vi "Load_Portfolio.vi"(7 "Config File path":path caption="Config File Path", 8 "error in (no error)":errorcluster caption="entrée d'erreur (pas d'erreur)", 11 "path":path) -> (0 "error out":errorcluster caption="sortie d'erreur", 3 "Portfolio en sortie":refnum<class "Portfolio.lvclass"> caption="DNL_LabVIEW Object out")   [LabVIEW 2012, in "Portfolio.lvclass"]
uses:
  Portfolio.lvclass
  Portfolio.lvclass/Portfolio.ctl
  Operation/Operation Parameters.ctl
  Operation/Operation Type Enum.ctl
  controls/Currencies.ctl
  Operation/Operation.lvclass
  Operation/Operation.lvclass/Operation.ctl
  Exchange/Exchange Parameters.ctl
  Exchange/Exchange Type Enum.ctl
  Exchange/Exchange.lvclass
  Exchange/Exchange.lvclass/Exchange.ctl
  Operations/Operations.lvclass
  Exchanges/Exchanges.lvclass
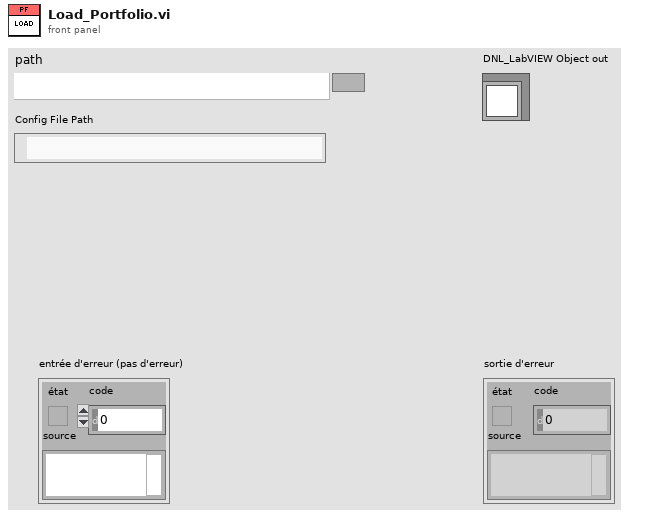
[diagram p1: front panel]
types:
  T1 = typedef "Portfolio Parameters.ctl" = cluster{"Date":timestamp, "Name":string, "Cash":dbl, "Total":dbl, "Investissements":dbl, "Performance Totale (en %)":dbl, "Performance sur 1 an (en %)":dbl}
  T2 = typedef "Operation Parameters.ctl" = cluster{"Date":timestamp, "Operation Type":T3, "Amount":dbl, "Comment":string, "Currency":T4}
  T3 = typedef "Operation Type Enum.ctl" = enum16{"Coupons", "Dépot", "Retrait", "Intérêts", "Taxe"}
  T4 = typedef "Currencies.ctl" = enum16{"Euro", "Dollar", "Yen", "RIM", "CHF"}
  T5 = typedef "Exchange Parameters.ctl" = cluster{"Date":timestamp, "Exchange Type":T6, "ISIN":string, "Label":string, "Price":dbl, "Qty":dbl, "Currency":T4, "Tax":dbl, "Comment":string, "PRU":dbl}
  T6 = typedef "Exchange.lvclass/Exchange Type Enum.ctl" = enum16{"ACHAT", "VENTE"}
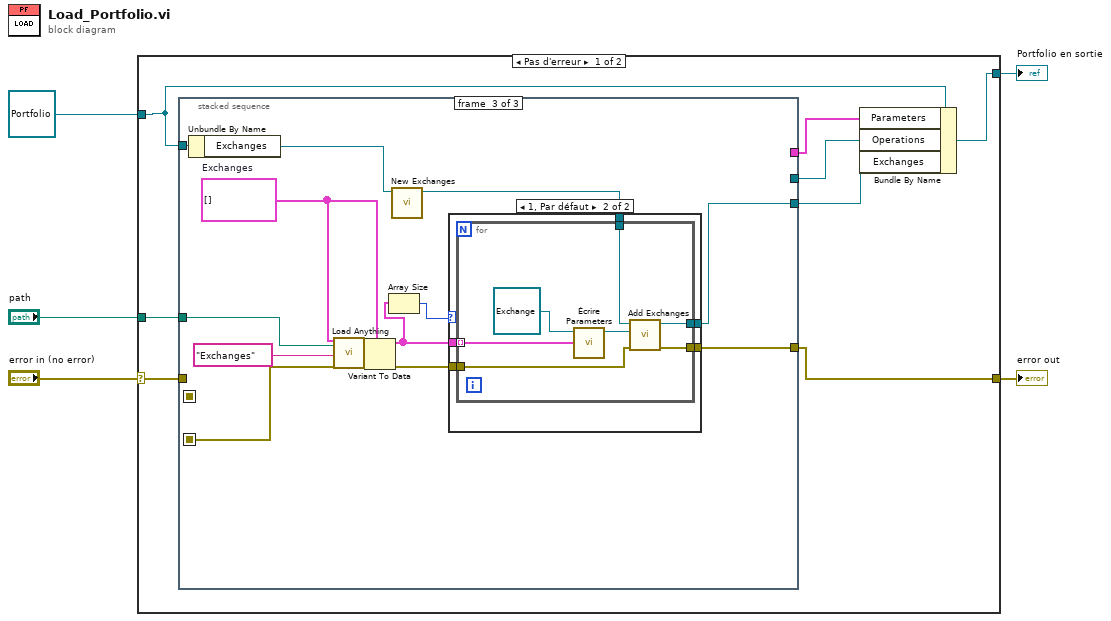
[diagram p0: block diagram]
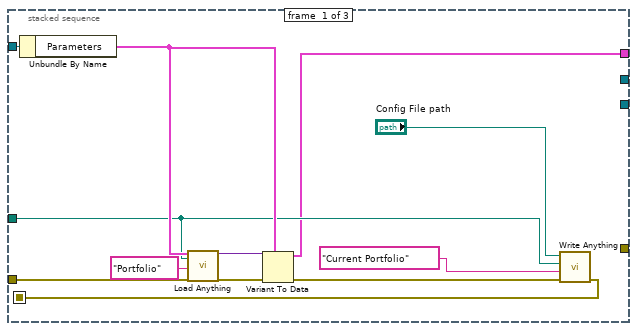
[diagram p2: hidden frame]
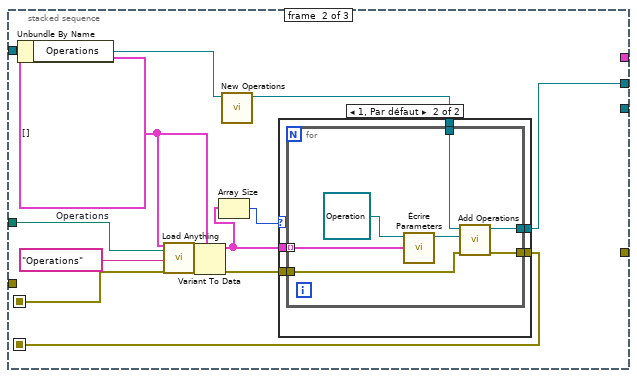
[diagram p3: hidden frame]
diagram:
  n1 = case shown="Pas d'erreur" "error in (no error)" {
    selector: "error in (no error)" -> [w13 w83]
    tunnel: [w11 w83] -> w4
    tunnel: [w9 w82] -> w2
    tunnel: refnum<class "Portfolio.lvclass"> refnum ("Portfolio en entrée") -> [w10 w82]
    tunnel: "path" -> [w12 _]
    frame No Error {
      n2 = stacked-sequence {
        seq-local: [w14 _ _] -> [_ w29 _]
        seq-local: [_ w26 _] -> [_ _ w56]
        tunnel: w10 -> [w25 w39 w67]
        tunnel: w13 -> [w22 _ _]
        tunnel: w12 -> [w17 w35 w63]
        tunnel: [_ _ w55] -> w11
        tunnel: [w15 _ _] -> w8
        tunnel: [_ w30 _] -> w7
        tunnel: [_ _ w54] -> w6
        frame #0 {
          n3 = Unbundle By Name(w25) -> ("Parameters"=w23:T1)
          n4 = call "Load Anything.vi"("Anything"=w23, "Path (dialog)"=w17, "Instance Name"="Portfolio", "Error In"=w22) -> ("Data"=w24:variant, "error out"=w21:errorcluster)  [unwired: 14 in]
          n5 = Variant To Data(error in=w21, type=w23, Variant=w24) -> (data=w15:T1, error out=w19:errorcluster)
          n6 = call "Write Anything.vi"("Error In"=w19, "Section Name (Name of \"Anything\")"="Current Portfolio" ("button label"), "Anything"=w17, "Path (dialog)"="Config File path") -> ("Error Out"=w14:errorcluster)  [unwired: 7 in]
        }
        frame #1 {
          w34 = T2[] []  # Operations
          n7 = Unbundle By Name(w39) -> ("Operations"=w32:refnum<class "Operations.lvclass">)
          n8 = call "Load Anything.vi"("Anything"=w34, "Path (dialog)"=w35, "Instance Name"="Operations", "Error In"=w29) -> ("Data"=w38:variant, "error out"=w37:errorcluster)  [unwired: 14 in]
          n9 = Variant To Data(error in=w37, type=w34, Variant=w38) -> (data=w28:T2[], error out=w33:errorcluster)
          n10 = Array Size(array=w28) -> (size(s)=w27:i32)
          n11 = call "New Operations.vi"("Operations en entrée"=w32) -> ("Operations en sortie"=w31:refnum<class "Operations.lvclass">)  [unwired: 9 in, 1 out]
          n12 = case shown="1, Par défaut" w27 {
            tunnel: w28 -> [_ w46]
            tunnel: w33 -> [w40 w45]
            tunnel: w31 -> [w41 w44]
            tunnel: [w40 w43] -> w26
            tunnel: [w41 w42] -> w30
            frame 0 {
            }
            frame 1, Default {
              n13 = for {
                tunnel: w46 -> [w52] mode=indexing
                tunnel: w45 -> [w48]
                tunnel: w44 -> [w51]
                tunnel: [w49] -> w42
                tunnel: [w47] -> w43
                n14 = call "Écrire Parameters.vi"("Parameters"=w52, "Operation en entrée"=refnum<class "Operation.lvclass"> refnum) -> ("Operation en sortie"=w50:refnum<class "Operation.lvclass">)  [unwired: 9 in]
                n15 = call "Add Operations.vi"("error in (no error)"=w48, "Added Operation"=w50, "Operations en entrée"=w51) -> ("error out"=w47:errorcluster, "Operations en sortie"=w49:refnum<class "Operations.lvclass">)  [unwired: 6 in, 1 out]
              }
            }
          }
        }
        frame #2 {
          w62 = T5[] []  # Exchanges
          n16 = Unbundle By Name(w67) -> ("Exchanges"=w60:refnum<class "Exchanges.lvclass">)
          n17 = call "Load Anything.vi"("Anything"=w62, "Path (dialog)"=w63, "Instance Name"="Exchanges", "Error In"=w56) -> ("Data"=w66:variant, "error out"=w65:errorcluster)  [unwired: 14 in]
          n18 = Variant To Data(error in=w65, type=w62, Variant=w66) -> (data=w58:T5[], error out=w61:errorcluster)
          n19 = Array Size(array=w58) -> (size(s)=w57:i32)
          n20 = call "New Exchanges.vi"("Exchanges en entrée"=w60) -> ("Exchanges en sortie"=w59:refnum<class "Exchanges.lvclass">)  [unwired: 9 in, 1 out]
          n21 = case shown="1, Par défaut" w57 {
            tunnel: w58 -> [_ w74]
            tunnel: w61 -> [w68 w73]
            tunnel: w59 -> [w69 w72]
            tunnel: [w68 w71] -> w55
            tunnel: [w69 w70] -> w54
            frame 0 {
            }
            frame 1, Default {
              n22 = for {
                tunnel: w74 -> [w80] mode=indexing
                tunnel: w73 -> [w76]
                tunnel: w72 -> [w79]
                tunnel: [w77] -> w70
                tunnel: [w75] -> w71
                n23 = call "Écrire Parameters.vi"("Parameters"=w80, "Exchange en entrée"=refnum<class "Exchange.lvclass"> refnum ("Operation en entrée")) -> ("Exchange en sortie"=w78:refnum<class "Exchange.lvclass">)  [unwired: 9 in]
                n24 = call "Add Exchanges.vi"("error in (no error)"=w76, "Exchange Added"=w78, "Exchanges en entrée"=w79) -> ("error out"=w75:errorcluster, "Exchanges en sortie"=w77:refnum<class "Exchanges.lvclass">)  [unwired: 6 in, 1 out]
              }
            }
          }
        }
      }
      n25 = Bundle By Name(cluster=w10, "Parameters"=w8, "Operations"=w7, "Exchanges"=w6) -> (w9:refnum<class "Portfolio.lvclass">)
    }
    frame Error {
    }
  }
  "error out" <- w4
  "Portfolio en sortie" <- w2
